vi "Add Type Specifier Constant to Frame.vi"(8 "error in (no error)":errorcluster, 10 "Frame In":refnum<vi>, 11 "Setter Generator In":refnum<class "Setter Generator.lvclass">) -> (0 "error out":errorcluster, 2 "Frame Out":refnum<vi>, 3 "Setter Generator Out":refnum<class "Setter Generator.lvclass">)   [LabVIEW 2020, in "Method Generation.lvlib" / "Setter Generator.lvclass"]
uses:
  Setter Generator.lvclass
  <vilib>/Utility/miscctls.llb/LVPointTypeDef.ctl
  Setter Generator.lvclass/Setter Generator.ctl
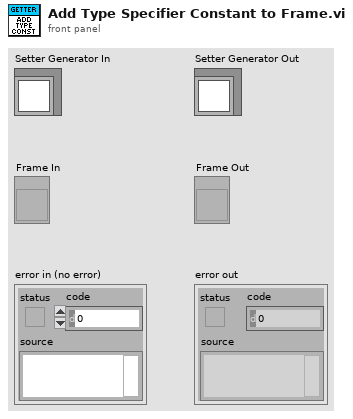
[diagram p1: front panel]
types:
  T1 = typedef "LVPointTypeDef.ctl" = cluster{"Horizontal":i16, "Vertical":i16}
  T2 = typedef "LVBoundsTypeDef.ctl" = cluster{"Width":u32, "Height":u32}
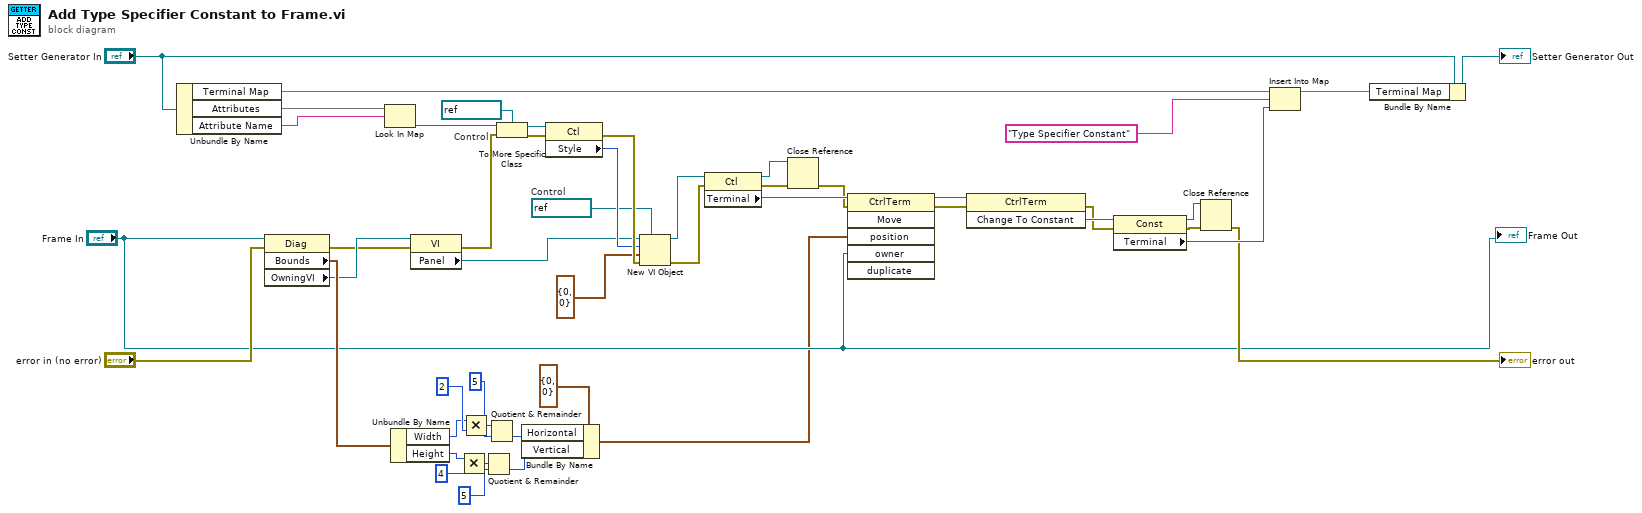
[diagram p0: block diagram]
diagram:
  w39 = refnum<vi> refnum  # Control
  w44 = refnum<vi> refnum  # Control
  n1 = Unbundle By Name("Setter Generator In") -> ("Terminal Map"=w29:map{string, refnum<vi>}, "Attributes"=w48:map{string, refnum<vi>}, "Attribute Name"=w47:string)
  n2 = property class="Diag"(reference="Frame In", error in="error in (no error)") -> (error out=w10:errorcluster, "Bounds"=w16:T2, "OwningVI"=w11:refnum<vi>)  [unwired: 1 out]
  n3 = Look In Map(map=w48, key=w47) -> (value=w42:refnum<vi>)  [unwired: 1 in, 1 out]
  n4 = Unbundle By Name(w16) -> ("Width"=w18:u32, "Height"=w25:u32)
  n5 = property class="VI"(reference=w11, error in=w10) -> (error out=w9:errorcluster, "Panel"=w8:refnum<vi>)  [unwired: 1 out]
  n6 = Multiply(x=w25, y=u32 4) -> (x*y=w14:u32)
  n7 = Multiply(x=w18, y=u32 2) -> (x*y=w20:u32)
  n8 = Quotient & Remainder(x=w14, y=i16 5 ("n")) -> (floor(x/y)=w22:u32)  [unwired: 1 out]
  n9 = Quotient & Remainder(x=w20, y=u32 5) -> (floor(x/y)=w23:u32)  [unwired: 1 out]
  n10 = To More Specific Class(target class=w44, reference=w42, error in=w9) -> (specific class reference=w45:refnum<vi>, error out=w43:errorcluster)
  n11 = Bundle By Name(cluster=T1 {"Horizontal"=0, "Vertical"=0} ("location"), "Horizontal"=w23, "Vertical"=w22) -> (w5:T1)
  n12 = property class="Ctl"(reference=w45, error in=w43) -> (error out=w41:errorcluster, "Style"=w40:u32)  [unwired: 1 out]
  n13 = New VI Object(vi object class=w39, owner refnum=w8, style=w40, position/next to=T1 {"Horizontal"=0, "Vertical"=0} ("location"), 8:w41) -> (object refnum=w32:refnum<vi>, 0:w12:errorcluster)  [unwired: 3 in]
  n14 = property class="Ctl"(reference=w32, error in=w12) -> (reference out=w34:refnum<vi>, error out=w38:errorcluster, "Terminal"=w4:refnum<vi>)
  n15 = Close Reference(reference=w34, error in (no error)=w38) -> (error out=w2:errorcluster)
  n16 = invoke class="CtrlTerm" method="Move"(reference=w4, error in=w2, "position"=w5, "owner"="Frame In") -> (reference out=w3:refnum<vi>, error out=w1:errorcluster)  [unwired: 2 in, 4 out]
  n17 = invoke class="CtrlTerm" method="Change To Constant"(reference=w3, error in=w1) -> (error out=w36:errorcluster, "Change To Constant"=w37:refnum<vi>)  [unwired: 1 in, 1 out]
  n18 = property class="Const"(reference=w37, error in=w36) -> (reference out=w33:refnum<vi>, error out=w35:errorcluster, "Terminal"=w27:refnum<vi>)
  n19 = Close Reference(reference=w33, error in (no error)=w35) -> (error out=→"error out":errorcluster)
  n20 = Insert Into Map(map in=w29, key="Type Specifier Constant", value=w27) -> (map out=w30:map{string, refnum<vi>})  [unwired: 2 out]
  n21 = Bundle By Name(cluster="Setter Generator In", "Terminal Map"=w30) -> (→"Setter Generator Out":refnum<class "Setter Generator.lvclass">)
  "Frame Out" <- "Frame In"
